vi "Subscribe to Events.vi"(8 "error in (no error)":errorcluster, 11 "Event Viewer Module in":refnum<class "Event Viewer Module.lvclass">) -> (0 "error out":errorcluster, 3 "Event Viewer Module out":refnum<class "Event Viewer Module.lvclass">)   [LabVIEW 2020, in "VolatusGUI.lvlib" / "Event Viewer Module.lvclass"]
uses:
  Event Viewer Module.lvclass
  C:/dev/lv20CE/relink/lv-volatus/Volatus/Module/Module.lvclass
  Volatus/Event Reporter Identity/Event Reporter Identity.lvclass
  C:/dev/lv20CE/relink/lv-volatus/Volatus/Identity/Identity.lvclass
  Volatus/Module/Module.lvclass/Module.ctl
  Volatus/MessageQ/MessageQ.lvclass/MessageQ.ctl
  Event Viewer Module.lvclass/Event Viewer Module.ctl
  Volatus/Module/Module.lvclass
  Volatus/VolatusAPI/VolatusAPI.lvclass
  Volatus/MessageQ/MessageQ.lvclass
  C:/dev/lv20CE/relink/lv-volatus/VolatusGUI/Event Viewer Module/Event Viewer Module.lvclass
  C:/dev/lv20CE/relink/lv-volatus/Volatus/Event Reporter Identity/Event Reporter Identity.lvclass
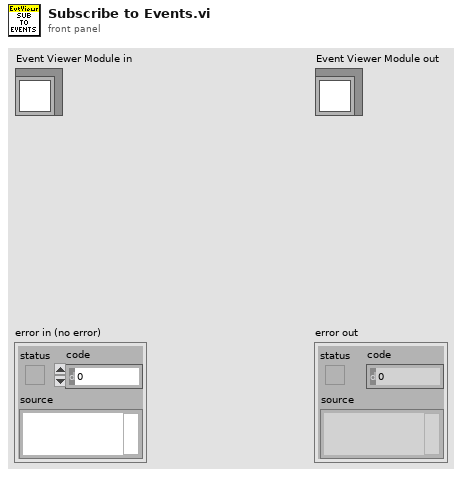
[diagram p1: front panel]
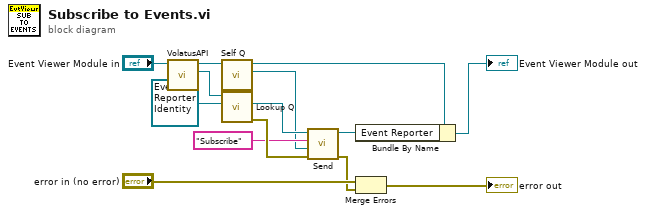
[diagram p0: block diagram]
diagram:
  n1 = call "VolatusAPI.vi"("Module in"="Event Viewer Module in") -> ("VolatusAPI"=w10:refnum<class "VolatusAPI.lvclass">, "Module out"=w11:refnum<class "Event Viewer Module.lvclass">)  [unwired: 9 in]
  n2 = call "Self Q.vi"("Module in"=w11) -> ("Self Q"=w5:refnum<class "MessageQ.lvclass">, "Module out"=w6:refnum<class "Event Viewer Module.lvclass">)  [unwired: 9 in]
  n3 = call "Lookup Q.vi"("Identity"=refnum<class "Event Reporter Identity.lvclass"> refnum ("Volatus:Event Reporter Identity.lvclass"), "VolatusAPI in"=w10) -> ("error out"=w14:errorcluster, "MessageQ"=w8:refnum<class "MessageQ.lvclass">)  [unwired: 7 in, 1 out]
  n4 = call "Send.vi"("error in (no error)"=w14, "Data"=w5, "ID"="Subscribe", "MessageQ in"=w8) -> ("error out"=w1:errorcluster, "MessageQ out"=w3:refnum<class "MessageQ.lvclass">)  [unwired: 6 in]
  n5 = Bundle By Name(cluster=w6, "Event Reporter"=w3) -> (→"Event Viewer Module out":refnum<class "Event Viewer Module.lvclass">)
  n6 = Merge Errors("error in (no error)", w1) -> (→"error out":errorcluster)
